vi "Create First Call Notifier.vi"(8 "error in (no error)":errorcluster, 11 "TwinCAT ADS in":refnum<class "TwinCAT ADS.lvclass">) -> (0 "error out":errorcluster, 3 "TwinCAT ADS out":refnum<class "TwinCAT ADS.lvclass">)   [LabVIEW 2018, in "TwinCAT ADS.lvclass"]
uses:
  TwinCAT ADS.lvclass
  TwinCAT ADS.lvclass/TwinCAT ADS.ctl
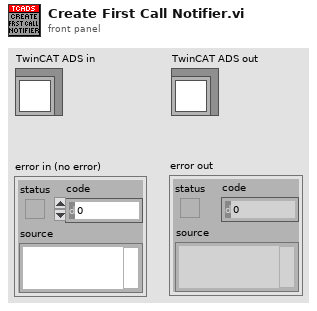
[diagram p1: front panel]
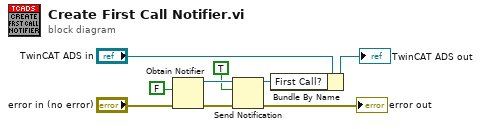
[diagram p0: block diagram]
diagram:
  n1 = Obtain Notifier(notification data type=FALSE, error in (no error)="error in (no error)") -> (notifier out=w9:refnum<notifier>, error out=w3:errorcluster)  [unwired: 2 in, 1 out]
  n2 = Send Notification(notification=TRUE, notifier=w9, error in (no error)=w3) -> (notifier out=w6:refnum<notifier>, error out=→"error out":errorcluster)
  n3 = Bundle By Name(cluster="TwinCAT ADS in", "First Call?"=w6) -> (→"TwinCAT ADS out":refnum<class "TwinCAT ADS.lvclass">)
